vi "List Class Hierarchies.vi"(8 "error in (no error)":errorcluster, 11 "Hierarchy Filter(empty=all)":string) -> (0 "error out":errorcluster, 1 "Success?":bool, 2 "Class Hierarchies":T1[](array[typedef]), 3 "Classes found":string[](array[string]))   [LabVIEW 2020, in "ClassLoader.lvlib"]
doc: "List class hierarchies. Can be filtered to only output Hierarchies that match Hierarchy Filter.\nThe last element in each hierarchy array is the class of that hierarchy.\n\nThis VI does not automatically load data. Front-load before calling this VI!"
uses:
  ClassLoader.lvlib
  Sub/Ctl/Ctl_Hierarchy Cluster.ctl
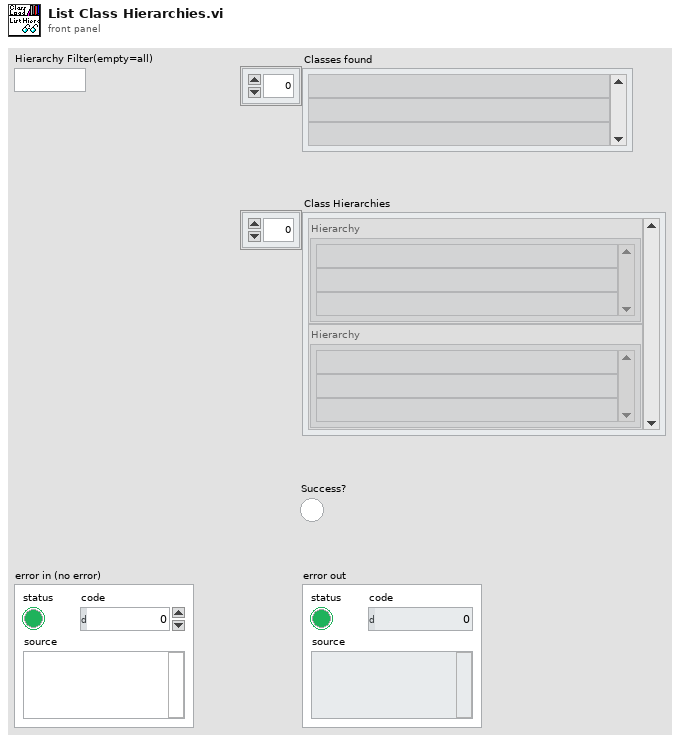
[diagram p1: front panel]
types:
  T1 = typedef "ClassLoader.lvlib/Ctl_Hierarchy Cluster.ctl" = cluster{"Hierarchy":string[]}
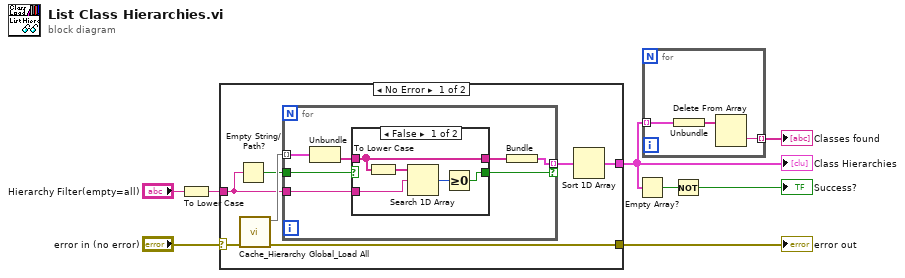
[diagram p0: block diagram]
diagram:
  n1 = To Lower Case(string="Hierarchy Filter(empty=all)") -> (all lower case string=w3:string)
  n2 = case shown="No Error" "error in (no error)" {
    selector: "error in (no error)" -> [w15 w30]
    tunnel: [w9 w30] -> w7
    tunnel: [w12 _] -> w2
    tunnel: w3 -> [w11 _]
    frame No Error {
      n3 = Empty String/Path?(string/path=w11) -> (empty?=w10:bool)
      n4 = call "Cache_Hierarchy Global_Load All.vi"("error in (no error)"=w15) -> ("error out"=w9:errorcluster, "Hierarchy Map"=w14:map{string, string[]})  [unwired: 8 in, 1 out]
      n5 = for {
        tunnel: w14 -> [w22] mode=indexing
        tunnel: [w21] -> w13 mode=indexing if=w20
        tunnel: w11 -> [w18]
        tunnel: w10 -> [w19]
        n6 = Unbundle(w22) -> ("value"=w17:string[])  [unwired: 1 out]
        n7 = case shown="False" w19 {
          selector: w19 -> [_ w29]
          tunnel: [w23 w29] -> w20
          tunnel: w18 -> [w25 _]
          tunnel: [w27 w28] -> w16
          tunnel: w17 -> [w27 w28]
          frame False {
            n8 = To Lower Case(string=w27) -> (all lower case string=w26:string[])
            n9 = Search 1D Array(1D array=w26, element=w25) -> (index of element=w24:i32)  [unwired: 1 in]
            n10 = Greater Or Equal To 0?(x=w24) -> (x >= 0?=w23:bool)
          }
          frame True {
          }
        }
        n11 = Bundle("value"=w16) -> (w21:cluster{"value":string[]})  [unwired: 1 in]
      }
      n12 = Sort 1D Array(array=w13) -> (sorted array=w12:cluster{"value":string[]}[])
    }
    frame Error {
    }
  }
  "error out" <- w7
  "Class Hierarchies" <- w2
  n13 = Empty Array?(array=w2) -> (empty?=w6:bool)
  n14 = for {
    tunnel: w2 -> [w33] mode=indexing
    tunnel: [w31] -> w1 mode=indexing
    n15 = Unbundle(w33) -> ("value"=w32:string[])
    n16 = Delete From Array(array=w32) -> (deleted portion=w31:string)  [unwired: 2 in, 1 out]
  }
  "Classes found" <- w1
  n17 = Not(x=w6) -> (.not. x?=→"Success?":bool)
